vi "Initialize.vi"(0 "FPGA I/O":refnum<k21>="Mod1/DIO0") -> (4 "BPT Ref":T1={"FPGA I/O"="Mod1/DIO0", "Buffer Ref"="", "Stop Ref"=""})   [LabVIEW 2016, in "UART 8N1 (FPGA).lvlib"]
uses:
  UART 8N1 (FPGA).lvlib
  UART Ref.ctl
  <vilib>/rvi/DataTransferAndStorage/Container/Common/niFpgaContainerGetUniqueNameForEmu.vi
  <vilib>/rvi/DataTransferAndStorage/Container/Common/niFpgaContainerSetEmuInfo.vi
  <vilib>/rvi/eio/common/nirviEmuReportErrorAndStop.vi
  <vilib>/rvi/DataTransferAndStorage/Container/Common/niFpgaContainerExecOnDevCompGetState.vi
  <vilib>/rvi/Emulation/niFpgaEmulationIsFPGAContextNoSignature.vi
  <vilib>/rvi/Memory/Memory_Emulation/niFpgaMemoryEmulationCacheClearOnFirstRun.vi
  <vilib>/rvi/Memory/Memory_Emulation/nirvimemoryEmulationManagerCache_MakeExclusive.vi
  <vilib>/rvi/Memory/Memory_Emulation/niFpgaMemoryEmulationValidateCache.vi
  <vilib>/rvi/Memory/Memory_Emulation/nirvimemoryEmulationManagerCache_InsertValue.vi
  <vilib>/Utility/error.llb/Clear Errors.vi
  <vilib>/rvi/Memory/Memory_Emulation/nirvimemoryEmulationManagerCache_ReleaseExclusive.vi
  <vilib>/rvi/Memory/Memory_Emulation/nirvimemoryEmulationManagerCache_GetValue.vi
  <vilib>/rvi/Memory/Memory_Emulation/nirvimemoryEmulationManagerCache_SetValue.vi
  <vilib>/rvi/Emulation/niFpgaProcessEmulError.vi
  <vilib>/rvi/Emulation/niFpgaSctlEmulationGetInTimedLoop.vi
  <vilib>/rvi/LocalResourceManager/LocalResourceManager.xnode
  <vilib>/rvi/DataTransferAndStorage/Container/XNode/niFpgaContainer.xnode
  <vilib>/rvi/DataTransferAndStorage/Register/Emulation/niFpgaRegisterEmulationRefIn.vi
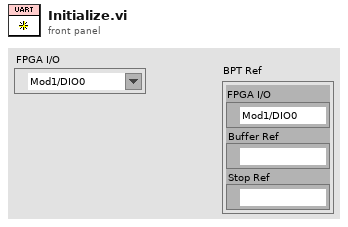
[diagram p1: front panel]
types:
  T1 = typedef "UART 8N1 (FPGA).lvlib/UART Ref.ctl" = cluster{"FPGA I/O":refnum<k21>, "Buffer Ref":refnum<k21>, "Stop Ref":refnum<k21>}
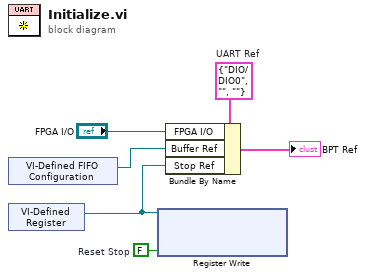
[diagram p0: block diagram]
diagram:
  w2 = FALSE  # Reset Stop
  w6 = T1 {"FPGA I/O"="DIO/DIO0", "Buffer Ref"="", "Stop Ref"=""}  # UART Ref
  n1 = xnode "VI-Defined FIFO Configuration"() -> ("FIFO Out"=w5:refnum<k21>)
  n2 = xnode "VI-Defined Register"() -> ("Register Out"=w3:refnum<k21>)
  n3 = xnode "Register Write"("Data"=w2, "Register In"=w3) -> ()  [unwired: 1 out]
  n4 = Bundle By Name(cluster=w6, "FPGA I/O"="FPGA I/O", "Buffer Ref"=w5, "Stop Ref"=w3) -> (→"BPT Ref":T1)
